vi "SwerveDrivePoseEst2_ResetPosition.vi"(6 "Pose":T10={"TRANSLATION"={"X"=0.0, "Y"=0.0}, "ROTATION"={"VALUE"=0.0, "COS"=1.0, "SIN"=0.0}} {"ROTATION"."SIN" format="%13.4f"; "ROTATION"."COS" format="%13.4f"; "ROTATION"."VALUE" format="%13.4f"; "TRANSLATION"."Y" format="%14.3f"; "TRANSLATION"."X" format="%14.3f"}, 9 "Module Positions":T1[](array[typedef]) {"Angle"."SIN" format="%13.4f"; "Angle"."COS" format="%13.4f"; "Angle"."VALUE" format="%13.4f"}, 10 "Gyro":T2={"VALUE"=0.0, "COS"=1.0, "SIN"=0.0} {"SIN" format="%13.4f"; "COS" format="%13.4f"; "VALUE" format="%13.4f"}, 11 "in SwerveDrivePoseEst2":T3={"M_Vision_K"=[], "m_nominal_dT"=0.0, "m_PrevTime_Sec"=0.0, "Pose_Buffer"={"TimeStamps"=[], "DataArray"=[], "Min_TimeStamp"=0.0, "Max_TimeStamp"=0.0, "ItemCount"=0, "MaxBufferTime"=0.0}, "Swerve_Drive_Kinematics"={"NumModules"=0, "InverseKinematics"=[], "ForwardKinematics"=[], "Modules"=[], "PrevCoR"={"X"=0.0, "Y"=0.0}, "SavedModuleStates"=[]}, "Swerve_Drive_Odom"={"POSE"={"TRANSLATION"={"X"=0.0, "Y"=0.0}, "ROTATION"={"VALUE"=0.0, "COS"=1.0, "SIN"=0.0}}, "GyroOffset"={"VALUE"=0.0, "COS"=1.0, "SIN"=0.0}, "PreviousAngle"={"VALUE"=0.0, "COS"=1.0, "SIN"=0.0}, "PrevModulePositions"=[], "NumModules"=0}, "M_Q"=[[0.0], [0.0], [0.0]], "NumModules"=-1} {"Swerve_Drive_Odom"."PrevModulePositions"."Angle"."SIN" format="%13.4f"; "Swerve_Drive_Odom"."PrevModulePositions"."Angle"."COS" format="%13.4f"; "Swerve_Drive_Odom"."PrevModulePositions"."Angle"."VALUE" format="%13.4f"; "Swerve_Drive_Odom"."PreviousAngle"."SIN" format="%13.4f"; "Swerve_Drive_Odom"."PreviousAngle"."COS" format="%13.4f"; "Swerve_Drive_Odom"."PreviousAngle"."VALUE" format="%13.4f"; "Swerve_Drive_Odom"."GyroOffset"."SIN" format="%13.4f"; "Swerve_Drive_Odom"."GyroOffset"."COS" format="%13.4f"; "Swerve_Drive_Odom"."GyroOffset"."VALUE" format="%13.4f"; "Swerve_Drive_Odom"."POSE"."ROTATION"."SIN" format="%13.4f"; "Swerve_Drive_Odom"."POSE"."ROTATION"."COS" format="%13.4f"; "Swerve_Drive_Odom"."POSE"."ROTATION"."VALUE" format="%13.4f"; "Swerve_Drive_Odom"."POSE"."TRANSLATION"."Y" format="%14.3f"; "Swerve_Drive_Odom"."POSE"."TRANSLATION"."X" format="%14.3f"; "Swerve_Drive_Kinematics"."SavedModuleStates"."Angle"."SIN" format="%13.4f"; "Swerve_Drive_Kinematics"."SavedModuleStates"."Angle"."COS" format="%13.4f"; "Swerve_Drive_Kinematics"."SavedModuleStates"."Angle"."VALUE" format="%13.4f"; "Swerve_Drive_Kinematics"."PrevCoR"."Y" format="%14.3f"; "Swerve_Drive_Kinematics"."PrevCoR"."X" format="%14.3f"; "Swerve_Drive_Kinematics"."Modules"."Y" format="%14.3f"; "Swerve_Drive_Kinematics"."Modules"."X" format="%14.3f"}) -> (3 "Out SwerveDrivePoseEst2":T3={"M_Vision_K"=[], "m_nominal_dT"=0.0, "m_PrevTime_Sec"=0.0, "Pose_Buffer"={"TimeStamps"=[], "DataArray"=[], "Min_TimeStamp"=0.0, "Max_TimeStamp"=0.0, "ItemCount"=0, "MaxBufferTime"=0.0}, "Swerve_Drive_Kinematics"={"NumModules"=0, "InverseKinematics"=[], "ForwardKinematics"=[], "Modules"=[], "PrevCoR"={"X"=0.0, "Y"=0.0}, "SavedModuleStates"=[]}, "Swerve_Drive_Odom"={"POSE"={"TRANSLATION"={"X"=0.0, "Y"=0.0}, "ROTATION"={"VALUE"=0.0, "COS"=1.0, "SIN"=0.0}}, "GyroOffset"={"VALUE"=0.0, "COS"=1.0, "SIN"=0.0}, "PreviousAngle"={"VALUE"=0.0, "COS"=1.0, "SIN"=0.0}, "PrevModulePositions"=[], "NumModules"=0}, "M_Q"=[[0.0], [0.0], [0.0]], "NumModules"=-1} {"Swerve_Drive_Odom"."PrevModulePositions"."Angle"."SIN" format="%13.4f"; "Swerve_Drive_Odom"."PrevModulePositions"."Angle"."COS" format="%13.4f"; "Swerve_Drive_Odom"."PrevModulePositions"."Angle"."VALUE" format="%13.4f"; "Swerve_Drive_Odom"."PreviousAngle"."SIN" format="%13.4f"; "Swerve_Drive_Odom"."PreviousAngle"."COS" format="%13.4f"; "Swerve_Drive_Odom"."PreviousAngle"."VALUE" format="%13.4f"; "Swerve_Drive_Odom"."GyroOffset"."SIN" format="%13.4f"; "Swerve_Drive_Odom"."GyroOffset"."COS" format="%13.4f"; "Swerve_Drive_Odom"."GyroOffset"."VALUE" format="%13.4f"; "Swerve_Drive_Odom"."POSE"."ROTATION"."SIN" format="%13.4f"; "Swerve_Drive_Odom"."POSE"."ROTATION"."COS" format="%13.4f"; "Swerve_Drive_Odom"."POSE"."ROTATION"."VALUE" format="%13.4f"; "Swerve_Drive_Odom"."POSE"."TRANSLATION"."Y" format="%14.3f"; "Swerve_Drive_Odom"."POSE"."TRANSLATION"."X" format="%14.3f"; "Swerve_Drive_Kinematics"."SavedModuleStates"."Angle"."SIN" format="%13.4f"; "Swerve_Drive_Kinematics"."SavedModuleStates"."Angle"."COS" format="%13.4f"; "Swerve_Drive_Kinematics"."SavedModuleStates"."Angle"."VALUE" format="%13.4f"; "Swerve_Drive_Kinematics"."PrevCoR"."Y" format="%14.3f"; "Swerve_Drive_Kinematics"."PrevCoR"."X" format="%14.3f"; "Swerve_Drive_Kinematics"."Modules"."Y" format="%14.3f"; "Swerve_Drive_Kinematics"."Modules"."X" format="%14.3f"})   [LabVIEW 2019, in "Trajectory_Library.lvlib"]
doc: "Resets the robot's position on the field.\n \nThe gyroscope angle does not need to be reset here on the user's robot code. The library automatically takes care of offsetting the gyro angle.\n \nInputs:\n - inSwerveDrvPoseEst2 -- SwerveDrvPoseEst2 -- Data cluster\n - gyroAngle -- Rotation2d -- The angle reported by the gyroscope.\n - ModulePositions -- ModulePositions -- The current module positions.\n - poseMeters -- Pose2d -- The position on the field that your robot is at.\n\nOutputs:\n - outSwerveDrvPoseEst2 -- SwerveDrvPoseEst2 -- Updated data cluster"
uses:
  Trajectory_Library.lvlib
  <vilib>/Analysis/Matrix/Datatypes/RealMatrix.ctl
  <vilib>/Analysis/Matrix/NI_Matrix.lvlib
  TypeDef/ROTATION2D.ctl
  TypeDef/TRANSLATION2D.ctl
  TypeDef/POSE2D.ctl
  TypeDef/TIME_INTERPOLATABLE_VARIANT.ctl
  TypeDef/SWERVE_DRIVE_MODULE_STATE.ctl
  TypeDef/SWERVE_DRIVE_KINEMATICS.ctl
  TypeDef/SWERVE_DRIVE_MODULE_POSITION.ctl
  TypeDef/SWERVE_DRIVE_ODOMETRY.ctl
  TypeDef/SWERVE_DRIVE_POSE_EST2.ctl
panel:
  # "<3, 1>"
  # "<3, 3>"
  # "<3, 1>"
  # "<3, 3>"
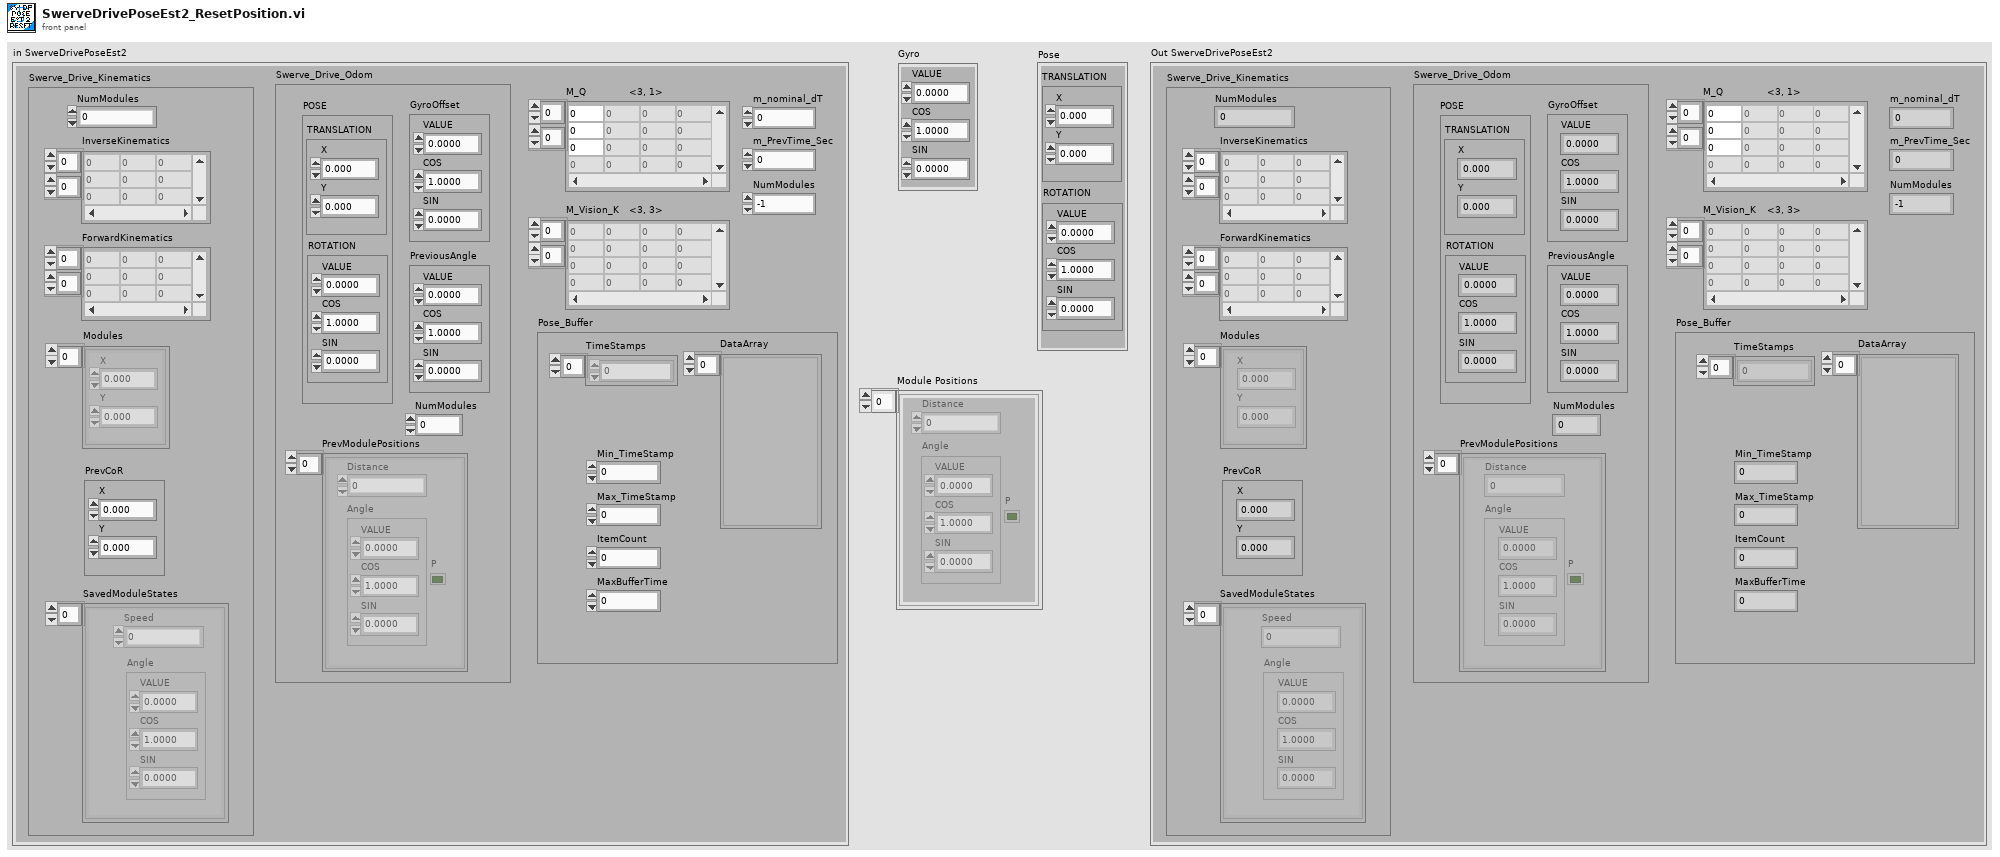
[diagram p1: front panel]
types:
  T1 = typedef "Trajectory_Library.lvlib/SWERVE_DRIVE_MODULE_POSITION.ctl" = cluster{"Distance":dbl, "Angle":T2, "P":bool}
  T2 = typedef "Trajectory_Library.lvlib/ROTATION2D.ctl" = cluster{"VALUE":dbl, "COS":dbl, "SIN":dbl}
  T3 = typedef "Trajectory_Library.lvlib/SWERVE_DRIVE_POSE_EST2.ctl" = cluster{"M_Vision_K":T4, "m_nominal_dT":dbl, "m_PrevTime_Sec":dbl, "Pose_Buffer":T5, "Swerve_Drive_Kinematics":T6, "Swerve_Drive_Odom":T9, "M_Q":T4, "NumModules":i32}
  T4 = typedef "NI_Matrix.lvlib/RealMatrix.ctl" = dbl[][]
  T5 = typedef "Trajectory_Library.lvlib/TIME_INTERPOLATABLE_VARIANT.ctl" = cluster{"TimeStamps":dbl[], "DataArray":variant[], "Min_TimeStamp":dbl, "Max_TimeStamp":dbl, "ItemCount":i32, "MaxBufferTime":dbl}
  T6 = typedef "Trajectory_Library.lvlib/SWERVE_DRIVE_KINEMATICS.ctl" = cluster{"NumModules":i32, "InverseKinematics":T4, "ForwardKinematics":T4, "Modules":T7[], "PrevCoR":T7, "SavedModuleStates":T8[]}
  T7 = typedef "Trajectory_Library.lvlib/TRANSLATION2D.ctl" = cluster{"X":dbl, "Y":dbl}
  T8 = typedef "Trajectory_Library.lvlib/SWERVE_DRIVE_MODULE_STATE.ctl" = cluster{"Speed":dbl, "Angle":T2}
  T9 = typedef "Trajectory_Library.lvlib/SWERVE_DRIVE_ODOMETRY.ctl" = cluster{"POSE":T10, "GyroOffset":T2, "PreviousAngle":T2, "PrevModulePositions":T1[], "NumModules":i32}
  T10 = typedef "Trajectory_Library.lvlib/POSE2D.ctl" = cluster{"TRANSLATION":T7, "ROTATION":T2}
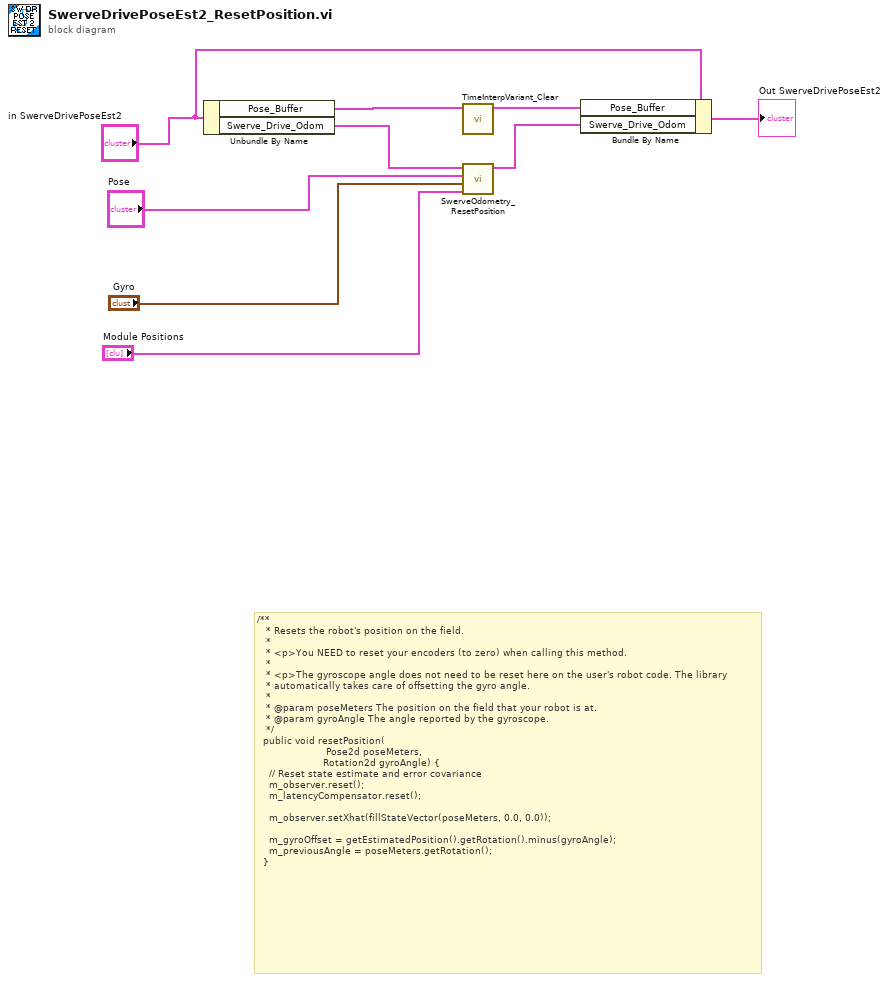
[diagram p0: block diagram]
diagram:
  # "/**\n   * Resets the robot's position on the field.\n   *\n   * <p>You NEED to reset your encoders (to zero) when calling this method.\n   *\n   * <p>The gyroscope angle does not need to be reset here on the user's robot code. The library\n   * automatically takes care of offsetting the gyro angle.\n   *\n   * @param poseMeters The position on the field that your robot is at.\n   * @param gyroAngle The angle reported by the gyroscope.\n   */\n  public void resetPosition(\n                       Pose2d poseMeters, \n                      Rotation2d gyroAngle) {\n    // Reset state estimate and error covariance\n    m_observer.reset();\n    m_latencyCompensator.reset();\n\n    m_observer.setXhat(fillStateVector(poseMeters, 0.0, 0.0));\n\n    m_gyroOffset = getEstimatedPosition().getRotation().minus(gyroAngle);\n    m_previousAngle = poseMeters.getRotation();\n  }"
  n1 = Unbundle By Name("in SwerveDrivePoseEst2") -> ("Pose_Buffer"=w8:T5, "Swerve_Drive_Odom"=w5:T9)
  n2 = call "TimeInterpVariant_Clear.vi"("in TimeInterpVariant"=w8) -> ("out TimeInterpVariant"=w7:T5)  [unwired: 10 in]
  n3 = call "SwerveOdometry_ResetPosition.vi"("Module Positions"="Module Positions", "gyroAngle"="Gyro", "Pose"="Pose", "in SWERVE_DRIVE_ODOMETRY"=w5) -> ("out SWERVE_DRIVE_ODOMETRY"=w4:T9)  [unwired: 6 in, 1 out]
  n4 = Bundle By Name(cluster="in SwerveDrivePoseEst2", "Pose_Buffer"=w7, "Swerve_Drive_Odom"=w4) -> (→"Out SwerveDrivePoseEst2":T3)
